vi "WaitAnswer.vi"(1 "VISA resource name in":refnum<visa-resource-name>) -> (0 "VISA resource name out":refnum<visa-resource-name>)   [LabVIEW 2016]
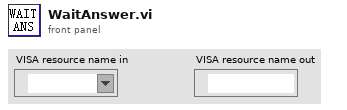
[diagram p1: front panel]
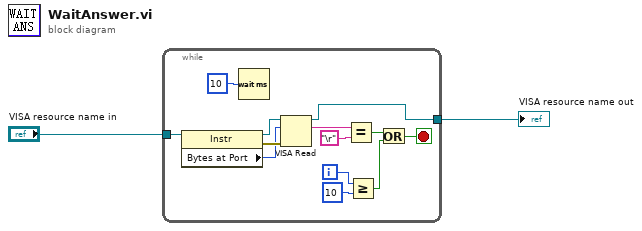
[diagram p0: block diagram]
diagram:
  n1 = while {
    tunnel: "VISA resource name in" -> [w10]
    tunnel: [w3] -> w1
    i -> [w14]
    stop <- w8 stop-if-true
    n2 = property class="Instr"(reference=w10) -> (reference out=w12:refnum<visa-resource-name>, error out=w11:errorcluster, "Bytes at Port"=w9:u32)  [unwired: 1 in]
    n3 = Wait (ms)(milliseconds to wait=u32 10 ("等待时间（毫秒）")) -> ()  [unwired: 1 out]
    n4 = VISA Read(VISA resource name=w12, byte count=w9, error in (no error)=w11) -> (VISA resource name out=w3:refnum<visa-resource-name>, read buffer=w7:string)  [unwired: 2 out]
    n5 = Equal?(x=w7, y="\r") -> (x = y?=w5:bool)
    n6 = Greater Or Equal?(x=w14, y=10) -> (x >= y?=w4:bool)
    n7 = Or(x=w5, y=w4) -> (x .or. y?=w8:bool)
  }
  "VISA resource name out" <- w1
